vi "GetElements(Multiple).vi"(7 "Qualified Name":string, 8 "error in (no error)":errorcluster, 10 "keys":string[](array[string]), 11 "ConfigManager in":refnum<class "ConfigManager.lvclass">) -> (0 "error out":errorcluster, 1 "Found":bool[](array[boolean]), 2 "Values":string[](array[string]), 3 "ConfigManager out":refnum<class "ConfigManager.lvclass">)   [LabVIEW 2013, in "CfgManager.lvlib" / "ConfigManager.lvclass"]
uses:
  ConfigManager.lvclass
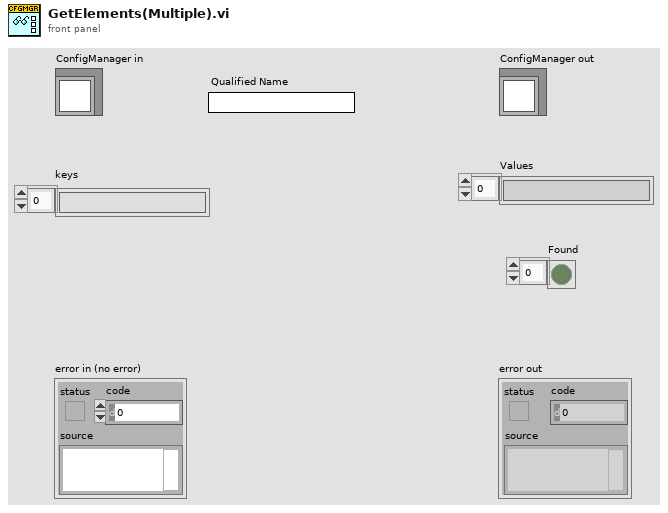
[diagram p1: front panel]
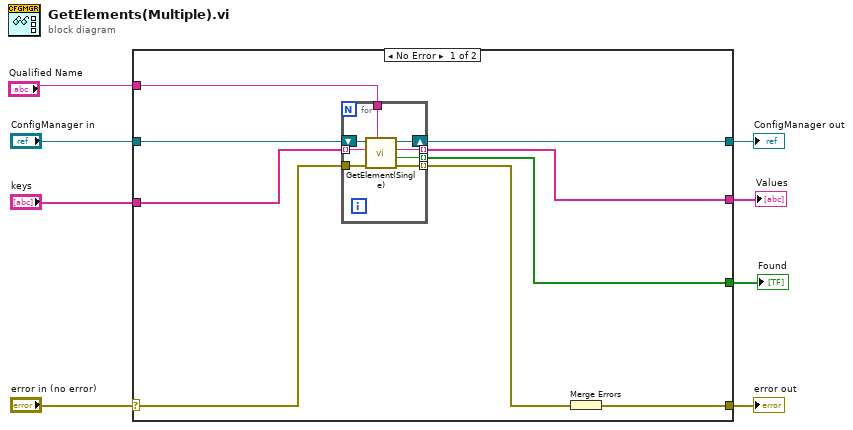
[diagram p0: block diagram]
diagram:
  n1 = case shown="No Error" "error in (no error)" {
    selector: "error in (no error)" -> [w13 w27]
    tunnel: [w11 w27] -> w7
    tunnel: [w16 w26] -> w5
    tunnel: "ConfigManager in" -> [w17 w26]
    tunnel: "keys" -> [w15 _]
    tunnel: [w14 _] -> w3
    tunnel: [w10 _] -> w2
    tunnel: "Qualified Name" -> [w9 _]
    frame No Error {
      n2 = for {
        tunnel: w15 -> [w23] mode=indexing
        tunnel: [w22] -> w14 mode=indexing
        tunnel: w13 -> [w21]
        tunnel: [w20] -> w12 mode=indexing
        shift-right: [w24] -> w16
        shift-left: w17 -> [w25]
        tunnel: [w19] -> w10 mode=indexing
        tunnel: w9 -> [w18]
        n3 = call-dynamic "GetElement(Single).vi"("Qualified Name"=w18, "error in (no error)"=w21, "Key"=w23, "ConfigManager in"=w25) -> ("error out"=w20:errorcluster, "found"=w19:bool, "Value"=w22:string, "ConfigManager out"=w24:refnum<class "ConfigManager.lvclass">)  [unwired: 4 in]
      }
      n4 = Merge Errors(w12) -> (w11:errorcluster)
    }
    frame Error {
    }
  }
  "error out" <- w7
  "ConfigManager out" <- w5
  "Values" <- w3
  "Found" <- w2
